vi "FP at the waypoint.vi"(0 "X of waypoint":dbl, 1 "Yof waypoint":dbl, 2 "Chase Mode?":bool, 3 "Y location":dbl, 4 "X location":dbl) -> (5 "At Waypoint?":bool)   [LabVIEW 2014]
doc: "This VI calculates the distance between the boat and a waypoint. If they are within 60 pixels the boat is at the waypoint. The output is Yes or No."
panel:
  in  "Radius":dbl=60.0 format="%#_13g"
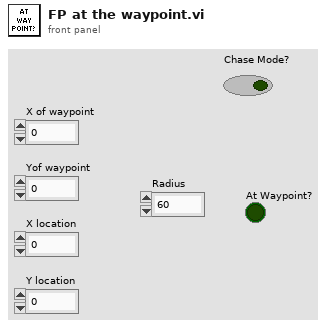
[diagram p1: front panel]
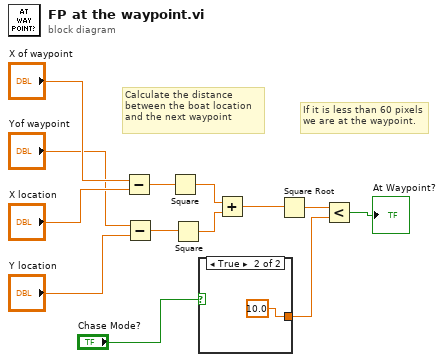
[diagram p0: block diagram]
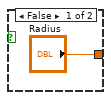
[diagram p2: hidden frame]
diagram:
  # "If it is less than 60 pixels\nwe are at the waypoint."
  # "Calculate the distance\nbetween the boat location\nand the next waypoint"
  n1 = Subtract(x="X of waypoint", y="X location") -> (x-y=w13:dbl)
  n2 = Subtract(x="Yof waypoint", y="Y location") -> (x-y=w12:dbl)
  n3 = Square(x=w13) -> (x^2=w11:dbl)
  n4 = Square(x=w12) -> (x^2=w10:dbl)
  n5 = case shown="True" "Chase Mode?" {
    tunnel: ["Radius" 10.0] -> w8
    frame False {
    }
    frame True {
    }
  }
  n6 = Add(x=w11, y=w10) -> (x+y=w2:dbl)
  n7 = Square Root(x=w2) -> (sqrt(x)=w9:dbl)
  n8 = Less?(x=w9, y=w8) -> (x < y?=→"At Waypoint?":bool)
